vi "loadDataToBuffer.vi"(8 "error in (no error)":errorcluster, 11 "niDAQmxAO in":refnum<class "niDAQmxAO.lvclass">) -> (0 "error out":errorcluster, 3 "niDAQmxAO out":refnum<class "niDAQmxAO.lvclass">)   [LabVIEW 2009, in "Hardware.lvlib" / "Channels.lvlib" / "niDAQmxAO.lvclass"]
uses:
  niDAQmxAO.lvclass
  <vilib>/DAQmx/write.llb/DAQmx Write (Analog 2D DBL NChan NSamp).vi
  AnalogOutput.lvclass
panel:
  out "Data":dbl[][](array[numeric])
  out "number of samples written per channel":u32
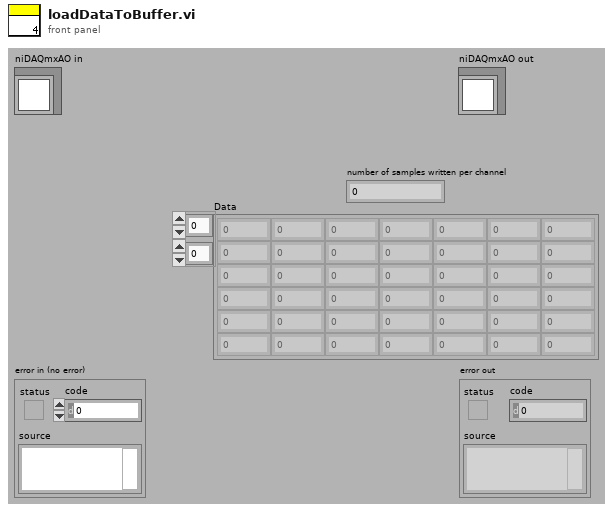
[diagram p1: front panel]
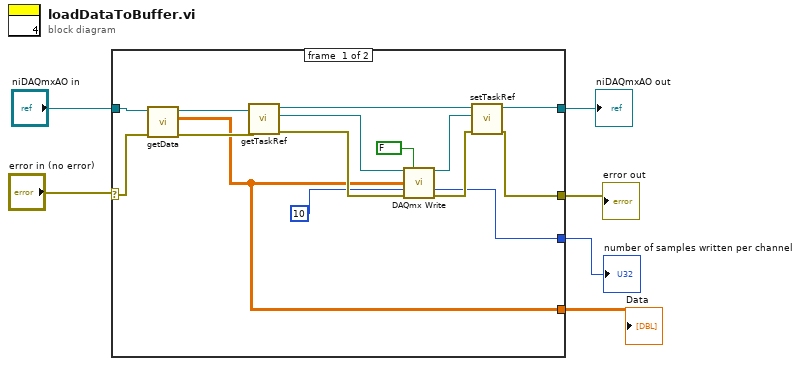
[diagram p0: block diagram]
diagram:
  n1 = case shown="No Error" "error in (no error)" {
    selector: "error in (no error)" -> [w20 w23]
    tunnel: [w12 w23] -> w5
    tunnel: [w13 w22] -> w3
    tunnel: "niDAQmxAO in" -> [w21 w22]
    tunnel: [w10 _] -> w2
    tunnel: [w8 _] -> w1
    frame #0 {
      n2 = call "getData.vi"("error in (no error)"=w20, "AnalogOutput.lvclass in"=w21) -> ("error out"=w18:errorcluster, "Data"=w8:dbl[][], "AnalogOutput.lvclass out"=w19:refnum<class "niDAQmxAO.lvclass">)  [unwired: 7 in]
      n3 = call "getTaskRef.vi"("error in (no error)"=w18, "niDAQmxAO.lvclass in"=w19) -> ("error out"=w17:errorcluster, "DAQmx Task Ref"=w7:refnum<k21>, "niDAQmxAO.lvclass out"=w15:refnum<class "niDAQmxAO.lvclass">)  [unwired: 7 in]
      n4 = call-poly <vilib>:"DAQmx Write.vi"("task/channels in"=w7, "auto start"=FALSE, "data"=w8, "timeout"=10, "error in"=w17) -> ("task out"=w16:refnum<k21>, "number of samples written per channel"=w10:u32, "error out"=w14:errorcluster)  [unwired: 8 in]
      n5 = call "setTaskRef.vi"("error in (no error)"=w14, "DAQmx Task Ref"=w16, "niDAQmxAO.lvclass in"=w15) -> ("error out"=w12:errorcluster, "niDAQmxAO.lvclass out"=w13:refnum<class "niDAQmxAO.lvclass">)  [unwired: 7 in]
    }
    frame #1 {
    }
  }
  "error out" <- w5
  "niDAQmxAO out" <- w3
  "number of samples written per channel" <- w2
  "Data" <- w1
